vi "SVT Integration (frequency).vi"   [LabVIEW 2017]
doc: "Converts acceleration to velocity or displacement. You can use this polymorphic VI to integrate a single spectrum or N spectra. The data type you wire to the <B>spectrum</B> input determines the polymorphic instance to use."
uses:
  <vilib>/addons/Sound and Vibration/svt_Integration/SoundVib_Integration.lvlib
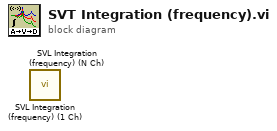
[diagram p0: block diagram]
diagram:
  n1 = call <vilib>:"SVL Integration (frequency) (1 Ch).vi"() -> ()  [unwired: 16 in, 4 out]
  n2 = call <vilib>:"SVL Integration (frequency) (N Ch).vi"() -> ()  [unwired: 16 in, 4 out]
